vi "close.vi"(8 "error IO":errorcluster) -> (0 "error":errorcluster)   [LabVIEW 2013, in "PicoMotor.lvclass"]
uses:
  PicoMotor.lvclass
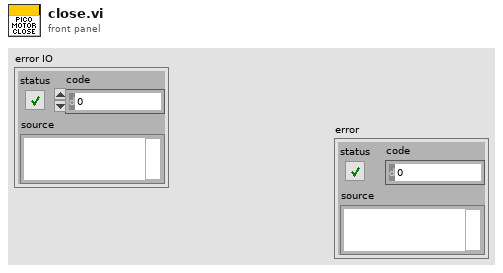
[diagram p1: front panel]
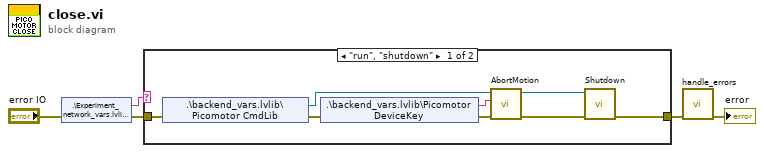
[diagram p0: block diagram]
diagram:
  n1 = shared-variable ".\\Experiment_network_vars.lvlib\\state"(error in="error IO") -> (w2:string, error out=w1:errorcluster)
  n2 = case shown="\"run\", \"shutdown\"" w2 {
    tunnel: [w11 w14] -> w5
    tunnel: w1 -> [w8 w14]
    frame "run", "shutdown" {
      n3 = shared-variable ".\\backend_vars.lvlib\\Picomotor CmdLib"(error in=w8) -> (w9:refnum<k24>, error out=w7:errorcluster)
      n4 = shared-variable ".\\backend_vars.lvlib\\Picomotor DeviceKey"(error in=w7) -> (w10:string, error out=w6:errorcluster)
      n5 = call "AbortMotion.vi"("error in (no error)"=w6, "DeviceKey In"=w10, "CmdLib In"=w9) -> ("error out"=w13:errorcluster, "CmdLib Out"=w12:refnum<k24>)  [unwired: 2 in, 1 out]
      n6 = call "Shutdown.vi"("error in (no error)"=w13, "CmdLib In"=w12) -> ("error out"=w11:errorcluster)  [unwired: 4 in, 1 out]
    }
    frame "halt", Default {
    }
  }
  n7 = call "handle_errors.vi"("error in (no error)"=w5) -> ("error out"=→"error":errorcluster)  [unwired: 10 in]
